vi "Read Grab Strenght.vi"(8 "Error In":errorcluster, 11 "Leap Handle In":T1) -> (0 "Error Out":errorcluster, 1 "Numeric Palm State":i32, 2 "Grab Strength":sgl, 3 "Leap Handle Out":T1, 5 "Palm State":string)   [LabVIEW 2014]
doc: "<b>Leap Read</b> requests and parses a <b>Frame</b> of data from the Leap Motion Controller. All the data associated with the Frame is organized into a LabVIEW cluster for accessibility.\n\nSpecifics about the data in the Frame cluster can be found by going to <b>Help » Leap Motion Controller Help</b> inside of LabVIEW"
uses:
  Typedef 2.0/Leap Handle.ctl
  C:/Users/Andrea/Desktop/Programmi LabView/Smart Wristband/Smart Wristband/Leap Motion VIs 2.0/LeapCSharp.NET4.0.dll
  LeapCSharp.NET4.0.dll
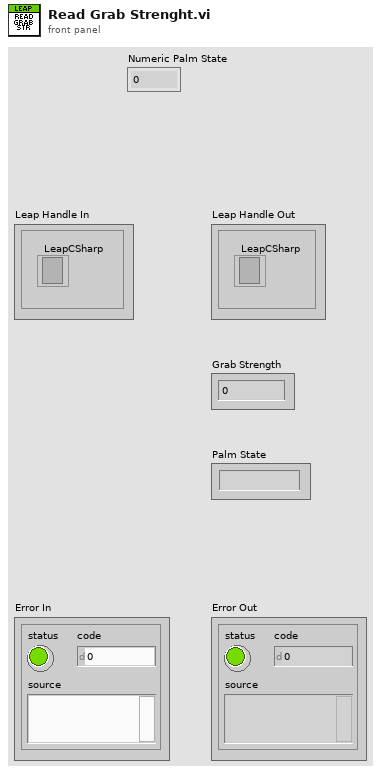
[diagram p1: front panel]
types:
  T1 = typedef "Leap Handle.ctl" = cluster{"LeapCSharp":refnum<k24>}
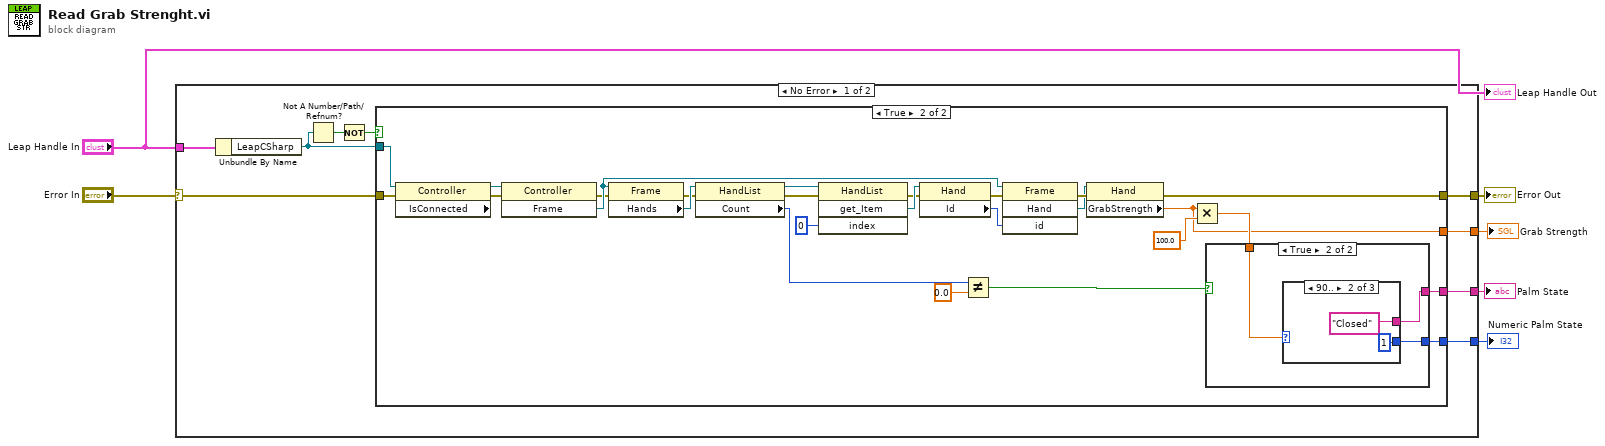
[diagram p0: block diagram]
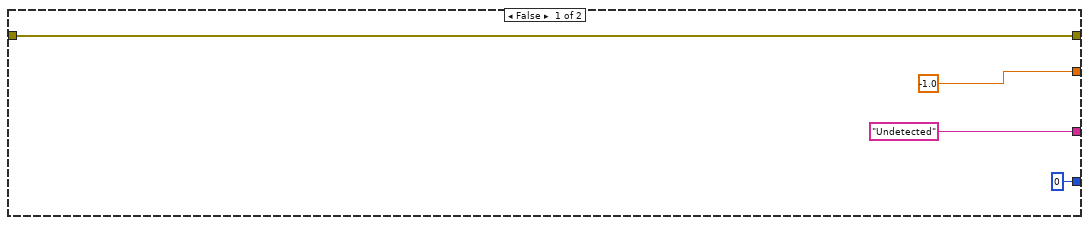
[diagram p2: hidden frame]
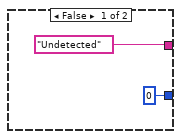
[diagram p3: hidden frame]
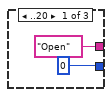
[diagram p4: hidden frame]
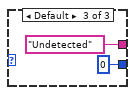
[diagram p5: hidden frame]
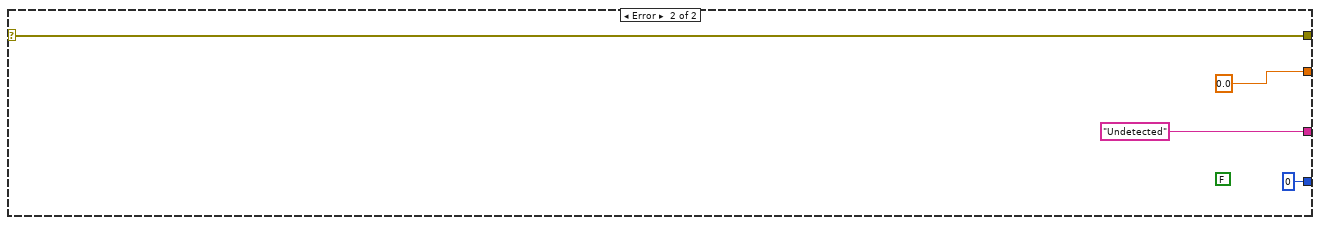
[diagram p6: hidden frame]
diagram:
  n1 = case shown="No Error" "Error In" {
    selector: "Error In" -> [w14 w60]
    tunnel: "Leap Handle In" -> [w15 _]
    tunnel: [w13 w60] -> w5
    tunnel: [w9 sgl 0.0 ("GrabStrength")] -> w3
    tunnel: [w8 "Undetected"] -> w2
    tunnel: [w7 0] -> w1
    frame No Error {
      n2 = Unbundle By Name(w15) -> ("LeapCSharp"=w10:refnum<k24>)
      n3 = Not A Number/Path/Refnum?(number/path/refnum=w10) -> (NaN/Path/Refnum?=w12:bool)
      n4 = Not(x=w12) -> (.not. x?=w11:bool)
      n5 = case shown="True" w11 {
        tunnel: w14 -> [w19 w45]
        tunnel: [w19 w28] -> w13
        tunnel: w10 -> [_ w42]
        tunnel: [sgl -1.0 ("GrabStrength") w21] -> w9
        tunnel: ["Undetected" w27] -> w8
        tunnel: [0 w20] -> w7
        frame False {
        }
        frame True {
          n6 = property class="Controller" props=["IsConnected"](reference=w42, error in=w45) -> (reference out=w44:refnum<k24>, error out=w43:errorcluster)  [unwired: 1 out]
          n7 = invoke class="Controller" method="Frame"(reference=w44, error in=w43) -> (error out=w33:errorcluster, "Frame"=w34:refnum<k24>)  [unwired: 1 in, 1 out]
          n8 = property class="Frame"(reference=w34, error in=w33) -> (error out=w32:errorcluster, "Hands"=w39:refnum<k24>)  [unwired: 1 out]
          n9 = property class="HandList"(reference=w39, error in=w32) -> (reference out=w38:refnum<k24>, error out=w31:errorcluster, "Count"=w23:i32)
          n10 = invoke class="HandList" method="get_Item"(reference=w38, error in=w31, "index"=0) -> (error out=w30:errorcluster, "get_Item"=w36:refnum<k24>)  [unwired: 1 in, 2 out]
          n11 = property class="Hand"(reference=w36, error in=w30) -> (error out=w29:errorcluster, "Id"=w35:i32)  [unwired: 1 out]
          n12 = Not Equal?(x=w23, y=0.0) -> (x != y?=w24:bool)
          n13 = invoke class="Frame" method="Hand"(reference=w34, error in=w29, "id"=w35) -> (error out=w41:errorcluster, "Hand"=w40:refnum<k24>)  [unwired: 1 in, 2 out]
          n14 = property class="Hand"(reference=w40, error in=w41) -> (error out=w28:errorcluster, "GrabStrength"=w21:sgl)  [unwired: 1 out]
          n15 = Multiply(x=w21, y=sgl 100.0) -> (x*y=w26:sgl)
          n16 = case shown="True" w24 {
            tunnel: ["Undetected" w50] -> w27
            tunnel: w26 -> [_ w49]
            tunnel: [0 w48] -> w20
            frame False {
            }
            frame True {
              n17 = case shown="90.." w49 {
                tunnel: ["Open" "Closed" "Undetected"] -> w50
                tunnel: [0 1 0] -> w48
                frame ..20 {
                }
                frame 90.. {
                }
                frame Default {
                }
              }
            }
          }
        }
      }
    }
    frame Error {
      (unwired) FALSE
    }
  }
  "Error Out" <- w5
  "Grab Strength" <- w3
  "Palm State" <- w2
  "Numeric Palm State" <- w1
  "Leap Handle Out" <- "Leap Handle In"
